vi "TEST - Replace Array Element.vi"(8 "error in (no error)":errorcluster) -> (0 "error out":errorcluster, 2 "pass":bool)   [LabVIEW 2020, in "test_openg_array.lvlib"]
uses:
  test_openg_array.lvlib
  <userlib>/_OpenG.lib/error/error.llb/openg_error.lvlib
  source/library/openg_variant.lvlib
panel:
  out "Failures":T1(array[cluster])
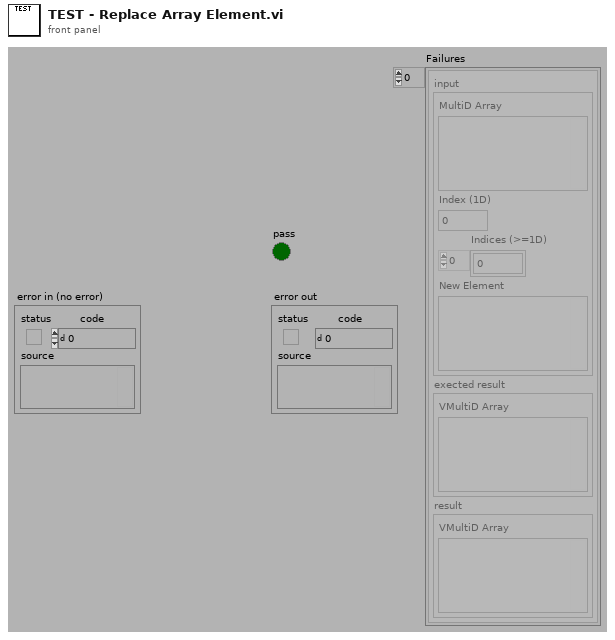
[diagram p1: front panel]
types:
  T1 = cluster{"input":cluster{"MultiD Array":variant, "Index (1D)":u32, "Indices (>=1D)":u32[], "New Element":variant}, "exected result":cluster{"VMultiD Array":variant}, "result":cluster{"VMultiD Array":variant}}[]
  T2 = cluster{"input":cluster{"MultiD Array":variant, "Index (1D)":u32, "Indices (>=1D)":u32[], "New Element":variant}, "exected result":cluster{"VMultiD Array":variant}, "result":cluster{"VMultiD Array":variant}}
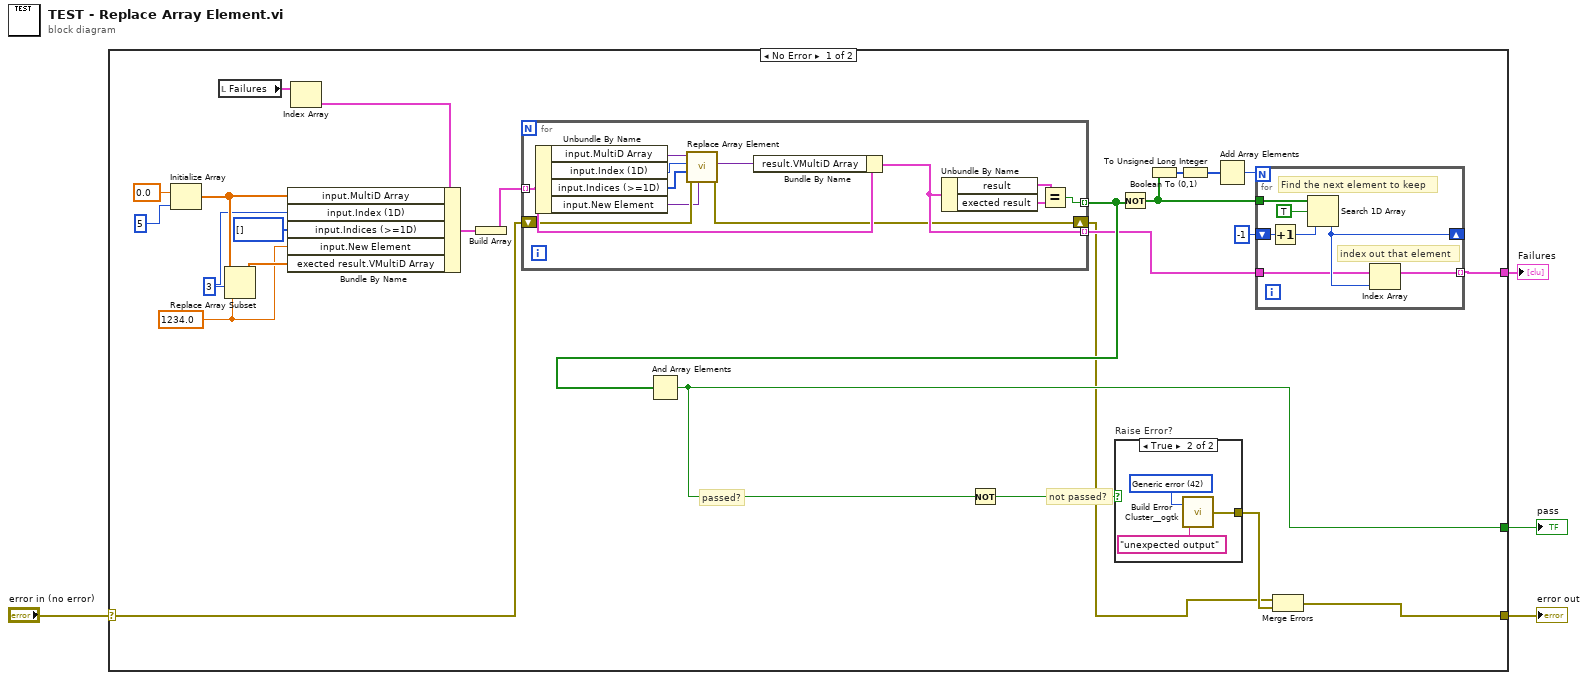
[diagram p0: block diagram]
diagram:
  n1 = case shown="No Error" "error in (no error)" {
    selector: "error in (no error)" -> [w15 w52]
    tunnel: [w26 _] -> w4
    tunnel: [w29 w52] -> w2
    tunnel: [w18 _] -> w1
    frame No Error {
      w7 = 1234.0 ("element")
      w6 = 3 ("index")
      # "not passed?"
      # "passed?"
      n2 = Initialize Array(0.0 ("element"), 5 ("dimension size")) -> (w9:dbl[])
      n3 = local read "Failures"() -> (w13:T1)
      n4 = Replace Array Subset(array=w9, new element=w7, index=w6) -> (w8:dbl[])
      n5 = Index Array(array=w13) -> (element=w12:T2)  [unwired: 1 in]
      n6 = Bundle By Name(cluster=w12, "input.MultiD Array"=w9, "input.Index (1D)"=w6, "input.Indices (>=1D)"=u32[] [], "input.New Element"=w7, "exected result.VMultiD Array"=w8) -> (w17:T2)
      n7 = Build Array(w17) -> (w16:T1)
      n8 = for {
        tunnel: w16 -> [w47] mode=indexing
        tunnel: [w48] -> w20 mode=indexing
        tunnel: [w46] -> w19 mode=indexing
        shift-right: [w42] -> w14
        shift-left: w15 -> [w41]
        n9 = Unbundle By Name(w47) -> ("input.MultiD Array"=w43:variant, "input.Index (1D)"=w39:u32, "input.Indices (>=1D)"=w38:u32[], "input.New Element"=w37:variant)
        n10 = call "Replace Array Element.vi"("New Element"=w37, "error in (no error)"=w41, "Indices (>=1D)"=w38, "Index (1D)"=w39, "MultiD Array"=w43) -> ("error out"=w42:errorcluster, "VMultiD Array"=w40:variant)  [unwired: 5 in]
        n11 = Bundle By Name(cluster=w47, "result.VMultiD Array"=w40) -> (w46:T2)
        n12 = Unbundle By Name(w46) -> ("result"=w45:cluster{"VMultiD Array":variant}, "exected result"=w44:cluster{"VMultiD Array":variant})
        n13 = Equal?(x=w45, y=w44) -> (x = y?=w48:bool)
      }
      n14 = And Array Elements(Boolean array=w20) -> (logical AND=w26:bool)
      n15 = Not(x=w26) -> (.not. x?=w27:bool)
      n16 = case "Raise Error?" shown="True" w27 {
        tunnel: [_ w49] -> w28
        frame False {
        }
        frame True {
          w50 = 42 items=["No error", "Argument error", "Memory is full", "Out of zone", "End of file", "File already open", "Generic file I/O error", "File not found", "File permission error", "Disk is full", "Duplicate path", "Too many files open", "System feature not enabled", "Resource file not found", "Cannot add resource", "Resource not found", "Image not found", "Image memory error", "Pen does not exist", "Config type invalid", "Config token not found", "Config parse error", "Config memory error", "Bad external code format", "Bad external code offset", "External code not present", "Null window", "Destroy window error", "Null menu", "Print aborted", "Bad print record", "Print driver error", "Windows error during printing", "Memory error during printing", "Print dialog error", "Generic print error", "Invalid device refnum", "Device not found", "Device parameter error", "Device unit error", "Cannot open device", "Device call aborted", "Generic error", "Cancelled by user", "Object ID too low", "Object ID too high", "Object not in heap", "Unknown heap", "Unknown object (invalid DefProc)", "Unknown object (DefProc not in table)", "Message out of range", "Invalid (null) method", "Unknown message", "Manager call not supported", "Bad address", "Network operation in progress", "Network operation timed out", "Connection is busy", "Network attribute not supported", "Network error", "Address in use", "System out of memory", "Connection aborted", "Connection refused", "Not connected", "Already connected", "Connection closed", "Initialization error (interapplication manager)", "Bad occurrence", "Wait on unbound occurrence handler", "Occurrence queue overflow", "Datalog type conflict", "Unused", "Unrecognized type (interapplication manager)", "Memory corrupt", "Failed to make temporary DLL", "Old CIN version", "Drag socket not found", "Failed to load drop-object", "Failed to register OLE object", "Failed to release OLE object", "Format specifier type mismatch", "Unknown format specifier", "Too few format specifiers", "Too many format specifiers", "Scan failed", "Newer CIN version", "Error converting to variant", "Runtime menu error", "Password tampered", "Variant attribute not found", "Incompatible variant data type", "Event data is not available", "Event Store is not present", "Occurrence is not found", "Event Queue is not created", "Event info is not available", "Refnum passed is NULL", "Error retrieving Class GUID", "Error retrieving CoClass GUID", "Error retrieving TypeLib GUID.", "Bad built application magic bytes.", "Specific driver is different from the specific driver associated with the Logical Name.", "There is no session opened to the class driver.", "Max Error", "MAX - Error with config objects", "MAX - Error loading configuration", "MAX - Group not supported"]
          n17 = call <userlib>:"Build Error Cluster__ogtk.vi"("String to Prepend to source (\"\")"="unexpected output" ("String to Prepend to source (\"\")"), "code"=w50) -> ("error out"=w49:errorcluster)
        }
      }
      n18 = Not(x=w20) -> (.not. x?=w22:bool[])
      n19 = Boolean To (0,1)(Boolean=w22) -> (0, 1=w23:i16[])
      n20 = To Unsigned Long Integer(number=w23) -> (unsigned 32bit integer=w21:u32[])
      n21 = Add Array Elements(numeric array=w21) -> (sum=w24:u32)
      n22 = for {
        N: w24 -> [_]
        tunnel: w19 -> [w32]
        tunnel: w22 -> [w36]
        shift-right: [w33] -> _
        shift-left: -1 ("start index (0)") -> [w34]
        tunnel: [w31] -> w18 mode=indexing
        # "index out that element"
        # "Find the next element to keep"
        n23 = Increment(x=w34) -> (x+1=w30:i32)
        n24 = Search 1D Array(1D array=w36, element=TRUE, start index (0)=w30) -> (index of element=w33:i32)
        n25 = Index Array(array=w32, index=w33) -> (element=w31:T2)
      }
      n26 = Merge Errors(w14, w28) -> (w29:errorcluster)
    }
    frame Error {
    }
  }
  "pass" <- w4
  "error out" <- w2
  "Failures" <- w1
